vi "TCL Get Base Signal.vi"(2 "error in (no error)":errorcluster, 3 "signal name":string, 4 "event number":i32) -> (0 "error out":errorcluster, 1 "signal":dbl[](array[numeric]))   [LabVIEW 2010]
doc: "This VI looks up the requested event number and then compares its rf frequency and modulation with the input values. If the event is found, and if the frequency and modulation match, the raw signal of the baseline is returned. Otherwise, an empty array is returned."
uses:
  TCL Global.vi
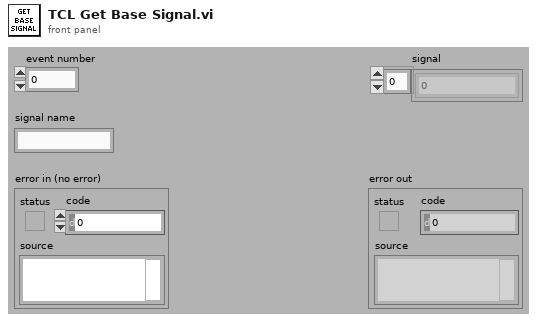
[diagram p1: front panel]
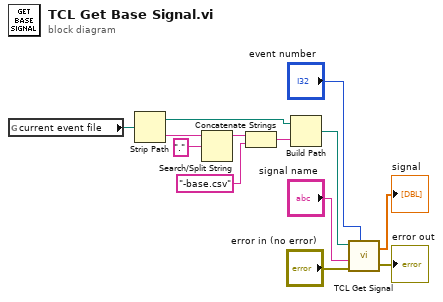
[diagram p0: block diagram]
diagram:
  n1 = global read "TCL Global.vi" "current event file"() -> (w8:path)
  n2 = Strip Path(path=w8) -> (stripped path=w1:path, name=w7:string)
  n3 = Search/Split String(string=w7, search string/char (-)=".") -> (substring before match=w5:string)  [unwired: 1 in, 2 out]
  n4 = Concatenate Strings(w5, "-base.csv" ("string")) -> (w2:string)
  n5 = Build Path(base path=w1, name or relative path=w2) -> (appended path=w3:path)
  n6 = call "TCL Get Signal.vi"("event number"="event number", "error in (no error)"="error in (no error)", "signal name"="signal name", "event file"=w3) -> ("error out"=→"error out":errorcluster, "signal"=→"signal":dbl[])  [unwired: 2 in]
